vi "SVT Unit Conversion.vi"   [LabVIEW 2017]
doc: "Converts between dB/linear, Magnitude/Magnitude^2, rms/peak/peak-peak, and dB ref1/dB ref2. You can use this polymorphic VI to convert a single spectrum, N spectra, one-channel complex spectrum, or N complex spectra. The data type you wire to the <B>spectrum</B> input determines the polymorphic instance to use."
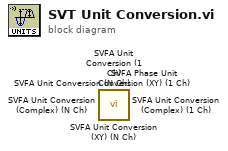
[diagram p0: block diagram]
diagram:
  n1 = call <vilib>:"SVFA Unit Conversion (XY) (N Ch).vi"() -> ()  [unwired: 16 in, 4 out]
  n2 = call <vilib>:"SVFA Phase Unit Conversion (XY) (1 Ch).vi"() -> ()  [unwired: 16 in, 4 out]
  n3 = call <vilib>:"SVFA Unit Conversion (Complex) (N Ch).vi"() -> ()  [unwired: 14 in, 6 out]
  n4 = call <vilib>:"SVFA Unit Conversion (Complex) (1 Ch).vi"() -> ()  [unwired: 14 in, 6 out]
  n5 = call <vilib>:"SVFA Unit Conversion (N Ch).vi"() -> ()  [unwired: 16 in, 4 out]
  n6 = call <vilib>:"SVFA Unit Conversion (1 Ch).vi"() -> ()  [unwired: 16 in, 4 out]
